vi "New2dBufferSizeCalc.vi"(6 "RowSize":u32, 8 "error in (no error)":errorcluster, 9 "new":u32, 10 "old":u32, 11 "Input":dbl[][](array[numeric])=[[nan, nan, nan, nan, nan, nan, nan], [nan, nan, nan, nan, nan, nan, nan], [nan, nan, nan, nan, nan, nan, nan], [nan, nan, nan, nan, nan, nan, nan], [nan, nan, nan, nan, nan, nan, nan], [nan, nan, nan, nan, nan, nan, nan], [nan, nan, nan, nan, nan, nan, nan], [nan, nan, nan, nan, nan, nan, nan], [nan, nan, nan, nan, nan, nan, nan], [nan, nan, nan, nan, nan, nan, nan]]) -> (0 "error out":errorcluster, 3 "Output":dbl[][](array[numeric]))   [LabVIEW 2015]
panel:
  out "y":i32
  out "Initialize 2D Array":dbl[][](array[numeric])
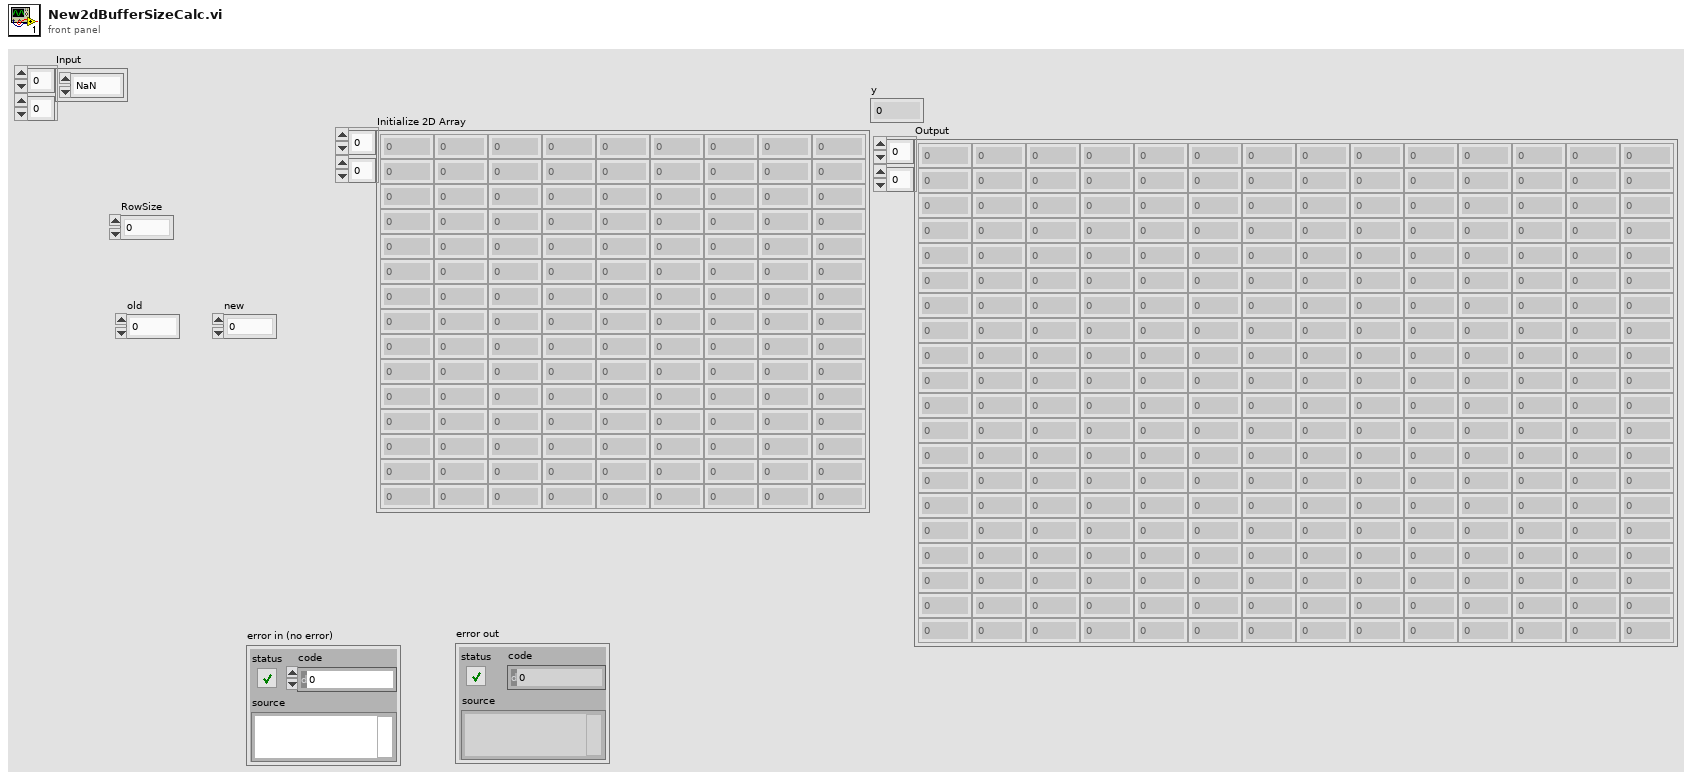
[diagram p1: front panel]
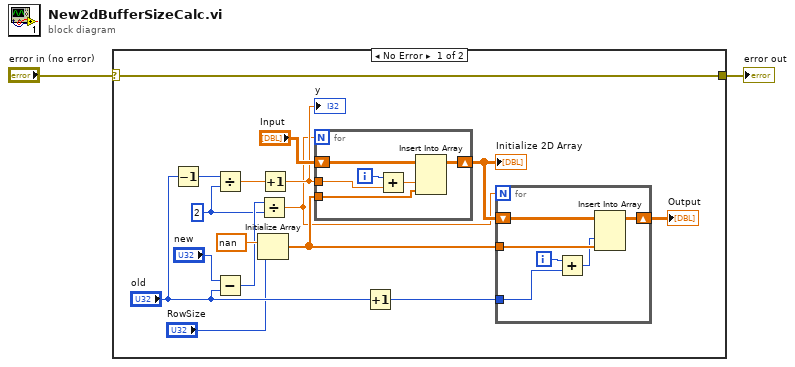
[diagram p0: block diagram]
diagram:
  n1 = case shown="No Error" "error in (no error)" {
    selector: "error in (no error)" -> [w4 w31]
    tunnel: [w4 w31] -> w1
    frame No Error {
      w13 = 2 ("y")
      n2 = Decrement(x="old") -> (x-1=w14:u32)
      n3 = Divide(x=w14, y=w13) -> (x/y=w12:dbl)
      n4 = Subtract(x="new", y="old") -> (x-y=w17:u32)
      n5 = Initialize Array(nan ("element"), "RowSize") -> (w8:dbl[])
      n6 = Divide(x=w17, y=w13) -> (x/y=w7:dbl)
      n7 = Increment(x=w12) -> (x+1=w11:dbl)
      "y" <- w11
      n8 = for {
        N: w7 -> [_]
        tunnel: w8 -> [w30]
        shift-right: [w29] -> w10
        shift-left: "Input" -> [w28]
        tunnel: w11 -> [w27]
        i -> [w25]
        n9 = Add(x=w25, y=w27) -> (x+y=w26:dbl)
        n10 = Insert Into Array(array=w28, index (col)=w26, new element=w30) -> (w29:dbl[][])  [unwired: 1 in]
      }
      "Initialize 2D Array" <- w10
      n11 = Increment(x="old") -> (x+1=w5:u32)
      n12 = for {
        N: w7 -> [_]
        tunnel: w8 -> [w24]
        shift-right: [w23] -> w9
        shift-left: w10 -> [w22]
        tunnel: w5 -> [w21]
        i -> [w19]
        n13 = Add(x=w19, y=w21) -> (x+y=w20:u32)
        n14 = Insert Into Array(array=w22, index (col)=w20, new element=w24) -> (w23:dbl[][])  [unwired: 1 in]
      }
      "Output" <- w9
    }
    frame Error {
    }
  }
  "error out" <- w1
